vi "GENser Config Local-Remote.vi"(7 "GEN Addr":i16=-1, 8 "error":errorcluster, 10 "Mode":enum16{"LOCAL", "REMOTE", "LOCKOUT"}(ring), 11 "VISA":refnum<visa-resource-name>) -> (0 "error out":errorcluster, 3 "VISA out":refnum<visa-resource-name>)   [LabVIEW 2017]
doc: "This VI sets the interface mode of the power supply. The input enumerated type may be:\n\n(0) LOCAL (Default). The power-supply settings are made from its front panel buttons and knobs \n(1) REMOTE. The power-supply settings are made using the serial port. The front panel may be used to view settings but not change them. The \"REM/LOC\" button may be pressed to set local mode\n(2) LOCKOUT. Same as Remote but the \"REM/LOC\" button will not operate to put the instrument into local mode\n\nNote: when in local mode, any serial command that changes the instrument's output state will put the instrument into remote mode"
panel:
  # "Lambda Genesys \n Serial Port\n  DC Power Supplies"
  # "Set Modes:\n Local, Remote, or Lockout"
  # "-1 = no address change"
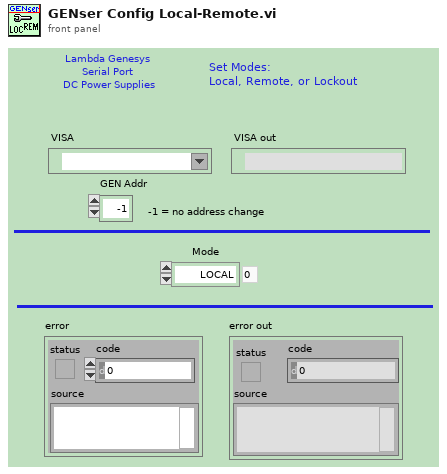
[diagram p1: front panel]
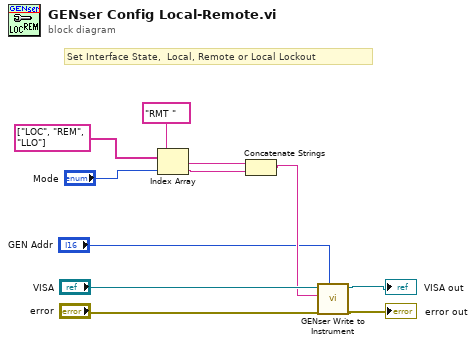
[diagram p0: block diagram]
diagram:
  # "Set Interface State,  Local, Remote or Local Lockout"
  n1 = Index Array(array=string[] ["LOC", "REM", "LLO"], index="Mode") -> (element=w4:string)
  n2 = Concatenate Strings("RMT ", w4) -> (w2:string)
  n3 = call "GENser Write to Instrument.vi"("GEN Addr"="GEN Addr", "error"="error", "Command"=w2, "VISA"="VISA") -> ("error out"=→"error out":errorcluster, "VISA out"=→"VISA out":refnum<visa-resource-name>)  [unwired: 5 in, 1 out]
